vi "CleanUpArray.vi"(0 "Ary In":string[][](array[string])) -> (17 "Count":dbl, 20 "Ary 1":string[](array[string]), 21 "Ary 2":string[](array[string]), 22 "Ary 3":string[](array[string]), 23 "Ary 4":string[](array[string]), 24 "Ary 5":string[](array[string]), 25 "Ary 6":string[](array[string]), 26 "Ary 7":string[](array[string]), 27 "Ary 8":string[](array[string]))   [LabVIEW 2018]
panel:
  out "size(s) 8":i32
  out "size(s) 7":i32
  out "size(s) 6":i32
  out "size(s) 5":i32
  out "size(s) 4":i32
  out "size(s) 3":i32
  out "size(s) 2":i32
  out "size(s)":i32
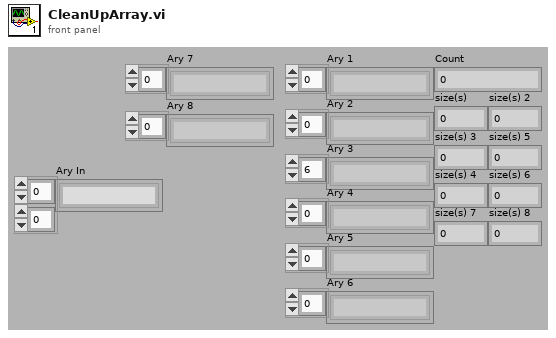
[diagram p1: front panel]
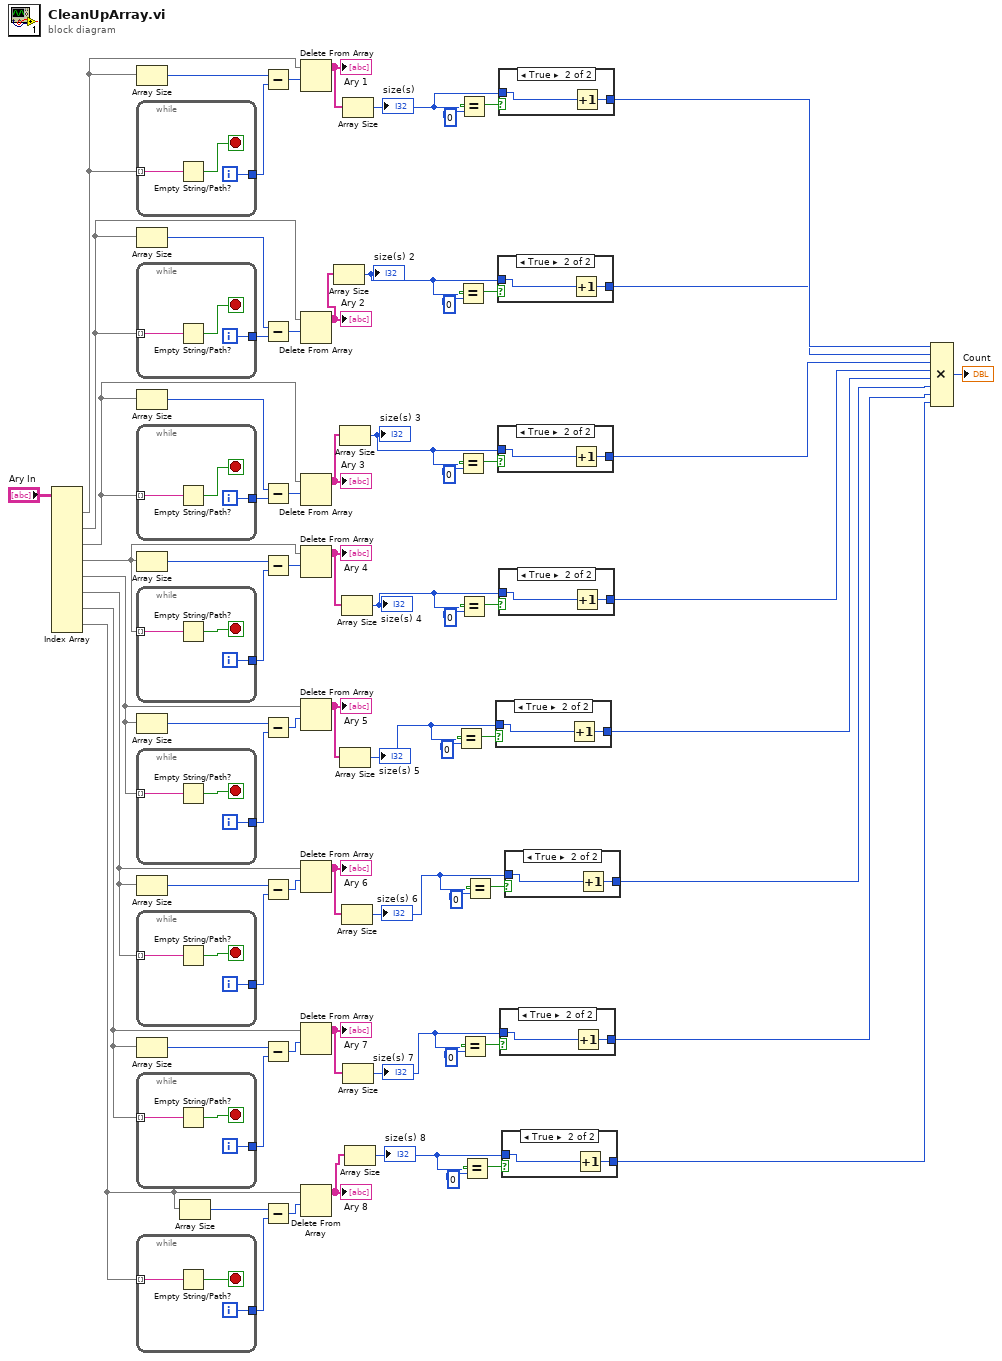
[diagram p0: block diagram]
diagram:
  n1 = Index Array(array="Ary In") -> (element #1=w70:string[], element #2=w66:string[], element #3=w62:string[], element #4=w58:string[], element #5=w54:string[], element #6=w50:string[], element #7=w46:string[], element #8=w42:string[])  [unwired: 16 in]
  n2 = Array Size(array=w70) -> (size(s)=w72:i32)
  n3 = while {
    tunnel: w70 -> [w77] mode=indexing
    tunnel: [w75] -> w73
    i -> [w75]
    stop <- w76 stop-if-true
    n4 = Empty String/Path?(string/path=w77) -> (empty?=w76:bool)
  }
  n5 = Array Size(array=w66) -> (size(s)=w67:i32)
  n6 = while {
    tunnel: w66 -> [w80] mode=indexing
    tunnel: [w78] -> w68
    i -> [w78]
    stop <- w79 stop-if-true
    n7 = Empty String/Path?(string/path=w80) -> (empty?=w79:bool)
  }
  n8 = Array Size(array=w62) -> (size(s)=w63:i32)
  n9 = while {
    tunnel: w62 -> [w83] mode=indexing
    tunnel: [w81] -> w64
    i -> [w81]
    stop <- w82 stop-if-true
    n10 = Empty String/Path?(string/path=w83) -> (empty?=w82:bool)
  }
  n11 = Array Size(array=w58) -> (size(s)=w59:i32)
  n12 = while {
    tunnel: w58 -> [w86] mode=indexing
    tunnel: [w84] -> w60
    i -> [w84]
    stop <- w85 stop-if-true
    n13 = Empty String/Path?(string/path=w86) -> (empty?=w85:bool)
  }
  n14 = Array Size(array=w54) -> (size(s)=w55:i32)
  n15 = while {
    tunnel: w54 -> [w89] mode=indexing
    tunnel: [w87] -> w56
    i -> [w87]
    stop <- w88 stop-if-true
    n16 = Empty String/Path?(string/path=w89) -> (empty?=w88:bool)
  }
  n17 = Array Size(array=w50) -> (size(s)=w51:i32)
  n18 = while {
    tunnel: w50 -> [w92] mode=indexing
    tunnel: [w90] -> w52
    i -> [w90]
    stop <- w91 stop-if-true
    n19 = Empty String/Path?(string/path=w92) -> (empty?=w91:bool)
  }
  n20 = Array Size(array=w46) -> (size(s)=w47:i32)
  n21 = while {
    tunnel: w46 -> [w95] mode=indexing
    tunnel: [w93] -> w48
    i -> [w93]
    stop <- w94 stop-if-true
    n22 = Empty String/Path?(string/path=w95) -> (empty?=w94:bool)
  }
  n23 = while {
    tunnel: w42 -> [w98] mode=indexing
    tunnel: [w96] -> w44
    i -> [w96]
    stop <- w97 stop-if-true
    n24 = Empty String/Path?(string/path=w98) -> (empty?=w97:bool)
  }
  n25 = Array Size(array=w42) -> (size(s)=w43:i32)
  n26 = Subtract(x=w72, y=w73) -> (x-y=w74:i32)
  n27 = Subtract(x=w67, y=w68) -> (x-y=w69:i32)
  n28 = Subtract(x=w63, y=w64) -> (x-y=w65:i32)
  n29 = Subtract(x=w59, y=w60) -> (x-y=w61:i32)
  n30 = Subtract(x=w55, y=w56) -> (x-y=w57:i32)
  n31 = Subtract(x=w51, y=w52) -> (x-y=w53:i32)
  n32 = Subtract(x=w47, y=w48) -> (x-y=w49:i32)
  n33 = Subtract(x=w43, y=w44) -> (x-y=w45:i32)
  n34 = Delete From Array(array=w70, length=w74) -> (array with subset deleted=w41:string[])  [unwired: 1 in, 1 out]
  "Ary 1" <- w41
  n35 = Delete From Array(array=w66, length=w69) -> (array with subset deleted=w40:string[])  [unwired: 1 in, 1 out]
  "Ary 2" <- w40
  n36 = Delete From Array(array=w62, length=w65) -> (array with subset deleted=w39:string[])  [unwired: 1 in, 1 out]
  "Ary 3" <- w39
  n37 = Delete From Array(array=w58, length=w61) -> (array with subset deleted=w38:string[])  [unwired: 1 in, 1 out]
  "Ary 4" <- w38
  n38 = Delete From Array(array=w54, length=w57) -> (array with subset deleted=w37:string[])  [unwired: 1 in, 1 out]
  "Ary 5" <- w37
  n39 = Delete From Array(array=w50, length=w53) -> (array with subset deleted=w36:string[])  [unwired: 1 in, 1 out]
  "Ary 6" <- w36
  n40 = Delete From Array(array=w46, length=w49) -> (array with subset deleted=w35:string[])  [unwired: 1 in, 1 out]
  "Ary 7" <- w35
  n41 = Delete From Array(array=w42, length=w45) -> (array with subset deleted=w34:string[])  [unwired: 1 in, 1 out]
  "Ary 8" <- w34
  n42 = Array Size(array=w40) -> (size(s)=w10:i32)
  "size(s) 2" <- w10
  n43 = Array Size(array=w39) -> (size(s)=w11:i32)
  "size(s) 3" <- w11
  n44 = Array Size(array=w37) -> (size(s)=w13:i32)
  "size(s) 5" <- w13
  n45 = Array Size(array=w38) -> (size(s)=w12:i32)
  "size(s) 4" <- w12
  n46 = Array Size(array=w36) -> (size(s)=w14:i32)
  "size(s) 6" <- w14
  n47 = Array Size(array=w41) -> (size(s)=w31:i32)
  "size(s)" <- w31
  n48 = Array Size(array=w35) -> (size(s)=w15:i32)
  "size(s) 7" <- w15
  n49 = Array Size(array=w34) -> (size(s)=w16:i32)
  "size(s) 8" <- w16
  n50 = Equal?(x=w13, y=0) -> (x = y?=w24:bool)
  n51 = Equal?(x=w10, y=0) -> (x = y?=w30:bool)
  n52 = Equal?(x=w11, y=0) -> (x = y?=w28:bool)
  n53 = Equal?(x=w31, y=0) -> (x = y?=w33:bool)
  n54 = Equal?(x=w12, y=0) -> (x = y?=w26:bool)
  n55 = Equal?(x=w15, y=0) -> (x = y?=w20:bool)
  n56 = Equal?(x=w16, y=0) -> (x = y?=w18:bool)
  n57 = Equal?(x=w14, y=0) -> (x = y?=w22:bool)
  n58 = case shown="True" w24 {
    tunnel: w13 -> [w99 w101]
    tunnel: [w99 w100] -> w5
    frame False {
    }
    frame True {
      n59 = Increment(x=w101) -> (x+1=w100:i32)
    }
  }
  n60 = case shown="True" w30 {
    tunnel: w10 -> [w102 w104]
    tunnel: [w102 w103] -> w8
    frame False {
    }
    frame True {
      n61 = Increment(x=w104) -> (x+1=w103:i32)
    }
  }
  n62 = case shown="True" w28 {
    tunnel: w11 -> [w105 w107]
    tunnel: [w105 w106] -> w7
    frame False {
    }
    frame True {
      n63 = Increment(x=w107) -> (x+1=w106:i32)
    }
  }
  n64 = case shown="True" w33 {
    tunnel: w31 -> [w108 w110]
    tunnel: [w108 w109] -> w9
    frame False {
    }
    frame True {
      n65 = Increment(x=w110) -> (x+1=w109:i32)
    }
  }
  n66 = case shown="True" w26 {
    tunnel: w12 -> [w111 w113]
    tunnel: [w111 w112] -> w6
    frame False {
    }
    frame True {
      n67 = Increment(x=w113) -> (x+1=w112:i32)
    }
  }
  n68 = case shown="True" w20 {
    tunnel: w15 -> [w114 w116]
    tunnel: [w114 w115] -> w3
    frame False {
    }
    frame True {
      n69 = Increment(x=w116) -> (x+1=w115:i32)
    }
  }
  n70 = case shown="True" w18 {
    tunnel: w16 -> [w117 w119]
    tunnel: [w117 w118] -> w2
    frame False {
    }
    frame True {
      n71 = Increment(x=w119) -> (x+1=w118:i32)
    }
  }
  n72 = case shown="True" w22 {
    tunnel: w14 -> [w120 w122]
    tunnel: [w120 w121] -> w4
    frame False {
    }
    frame True {
      n73 = Increment(x=w122) -> (x+1=w121:i32)
    }
  }
  n74 = Compound Arithmetic op=MULTIPLY(w9, w8, w7, w6, w5, w4, w3, w2) -> (→"Count":i32)
